vi "Durability_will_2012_07_05.vi"() -> ()   [LabVIEW 2011]
uses:
  <vilib>/DAQmx/write.llb/DAQmx Write (Counter Time 1Chan 1Samp).vi
  <vilib>/DAQmx/read.llb/DAQmx Read (Analog 1D Wfm NChan NSamp).vi
  <vilib>/measure/madcrms.llb/Basic Averaged DC-RMS for 1 Chan.vi
  <vilib>/DAQmx/miscellaneous.llb/DAQmx Fill In Error Info.vi
  <vilib>/Analysis/NI_AALBase.lvlib
  <vilib>/measure/NI_MAPro.lvlib
panel:
  out "Positive Peak":dynamicdata(graph)
  out "Negative Peak":dynamicdata(graph)
  out "Motor 1 Elapsed Time (s)":string caption="Elapsed Time Text"
  out "Motor 1 Start Time":string caption="Start Time Text"
  out "Motor 1 Down":bool
  out "Long Write":bool caption="Time has Elapsed"
  out "Short Write":bool caption="Time has Elapsed"
  out "Temps":dynamicdata(graph) caption="Signal Out"
  out "Power Graph":dynamicdata(graph) caption="Collected Signals"
  out "Errors":errorcluster
  out "RPM":dynamicdata(graph) caption="Collected Signals"
  out "Motor RPM":dbl format="%#.0f"
  out "Motor Power (watts)":dbl format="%#.4f"
  out "Power to MC1 (watts)":dbl format="%#.4f"
  out "Voltage to MC1 (volts)":dbl format="%#.4f"
  out "Current to MC1  (amps)":dbl format="%#.4f"
  in  "Manual Start":bool
  in  "Power \nSetting":i8(slide) min=0 max=100 step=10 scale=0.0..100.0
  out "Power Setting (%)":dbl format="%#.2f"
  out "Motor Temp (F)":dbl format="%.1f"
  out "Tank Temp (F)":dbl format="%.1f"
  in  "Quit 4":bool
  out "Phase to Phase Voltage":waveform(dbl)(graph)
  out "Phase Current":waveform(dbl)(graph)
  # "Temperature"
  # "MC1"
  # "Motor Power and RPM"
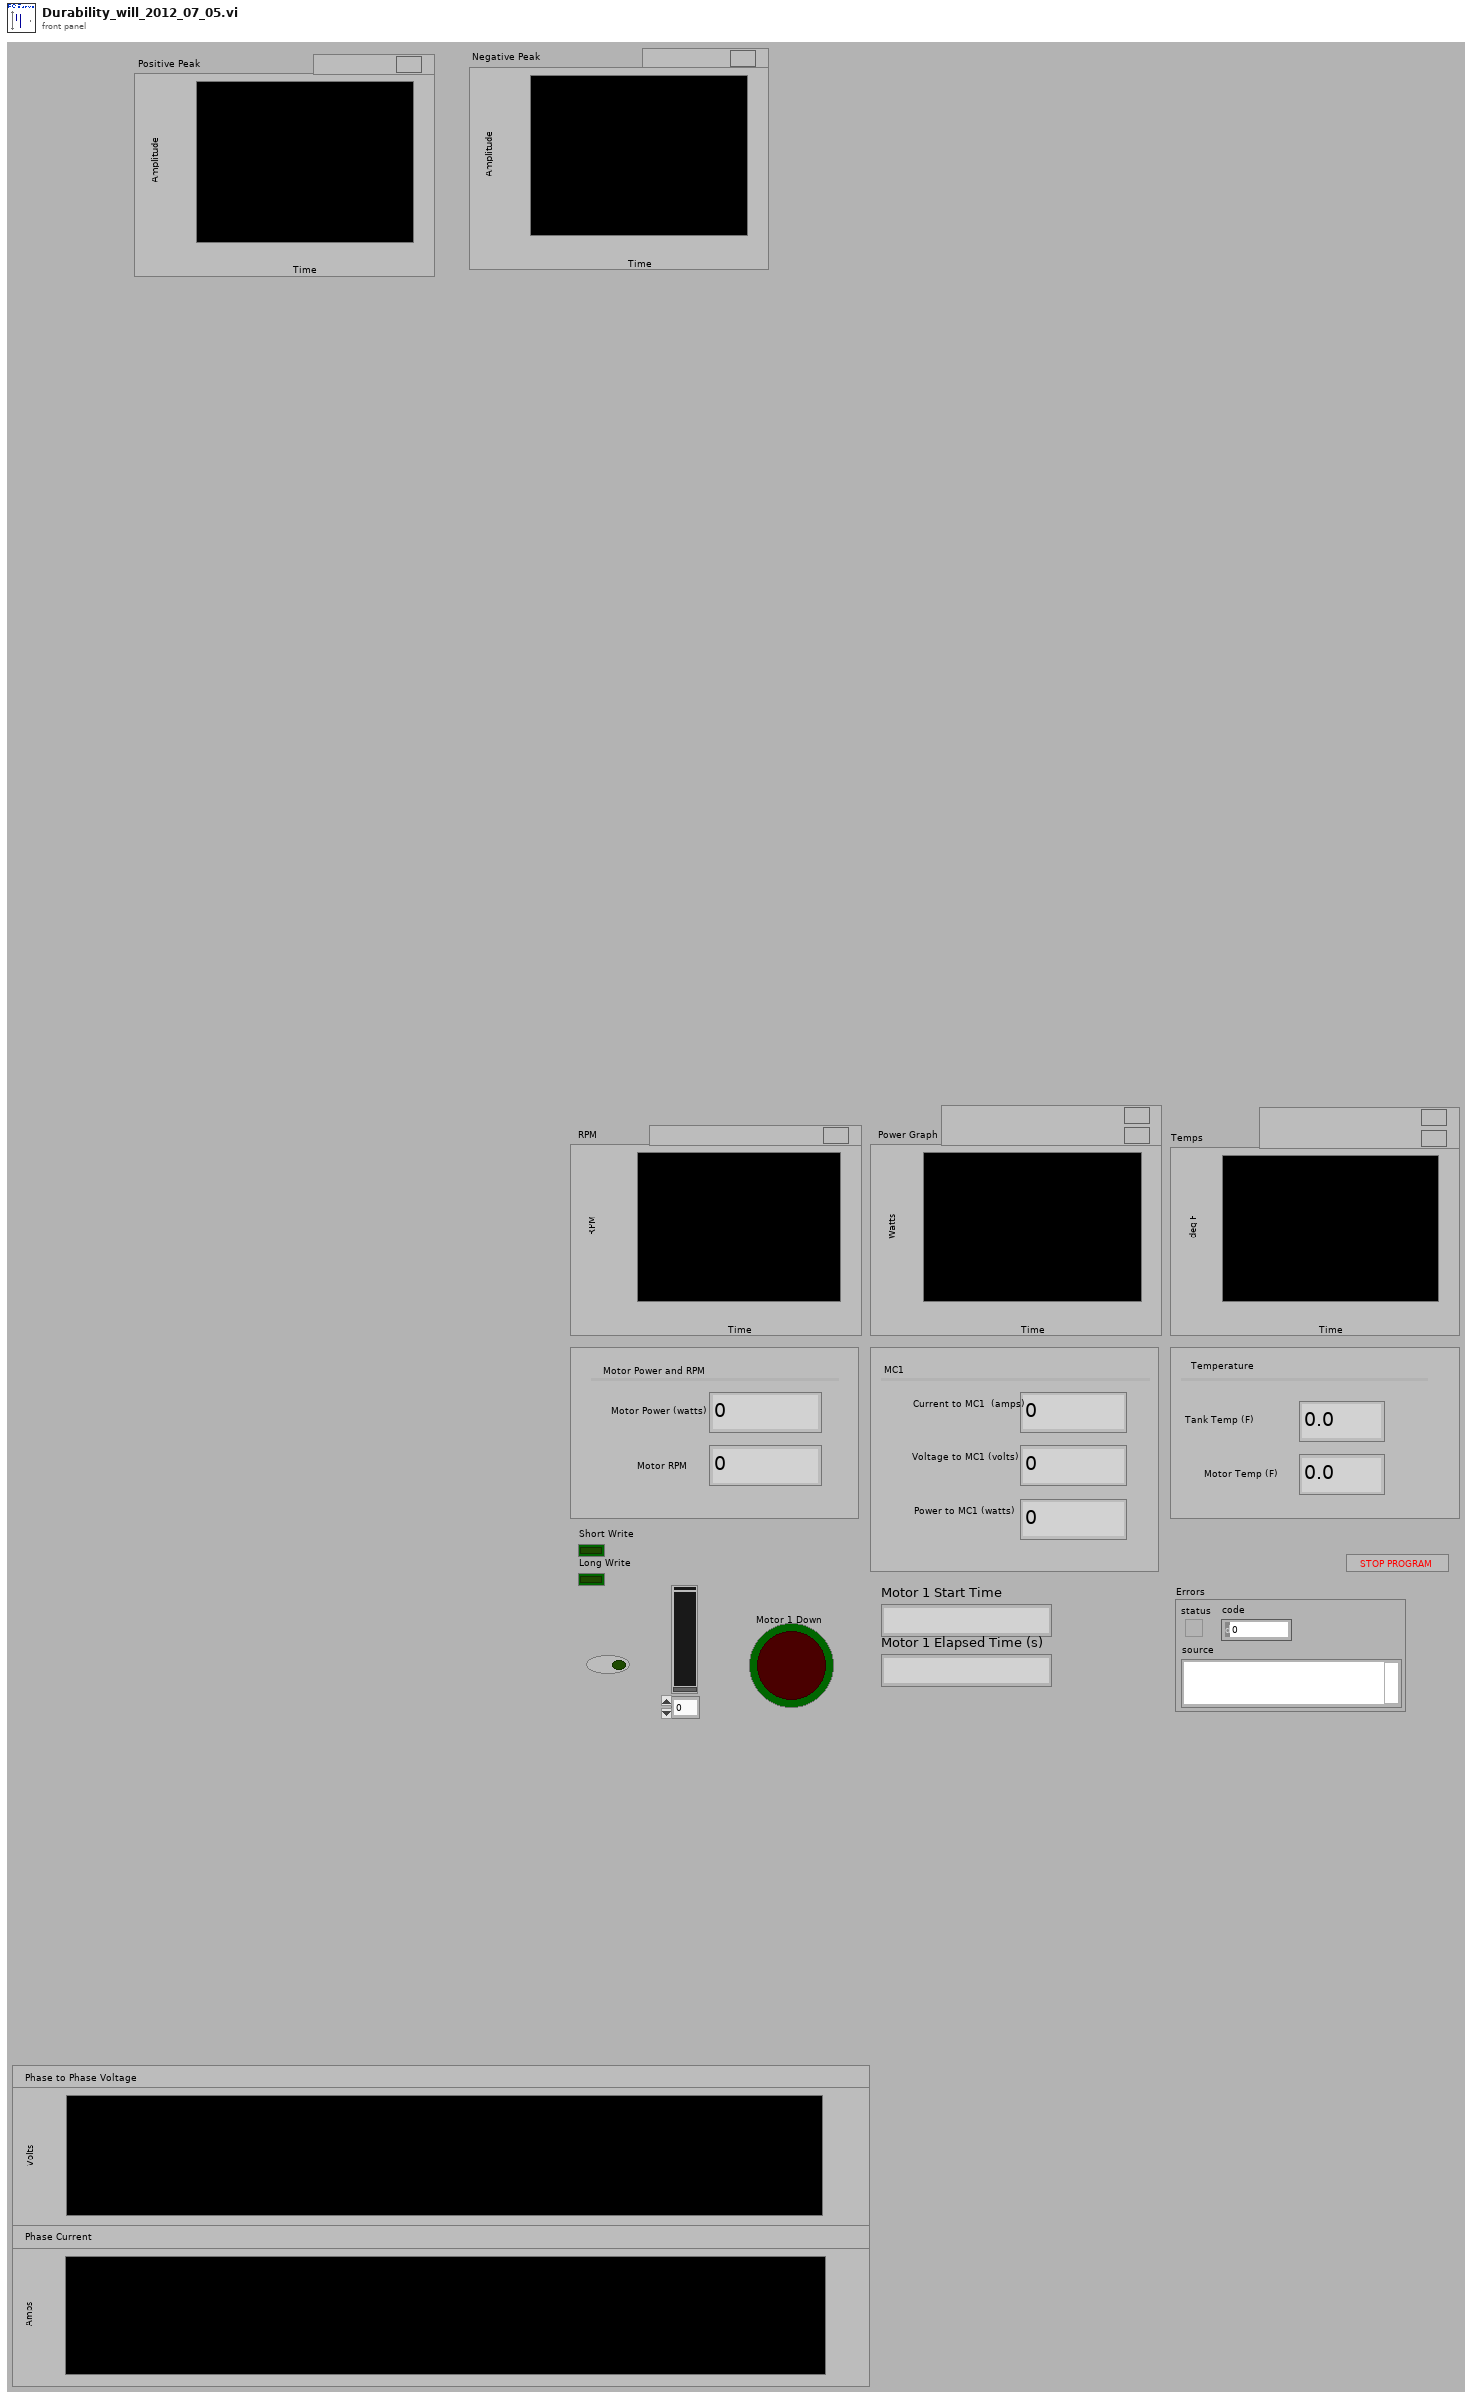
[diagram p1: front panel]
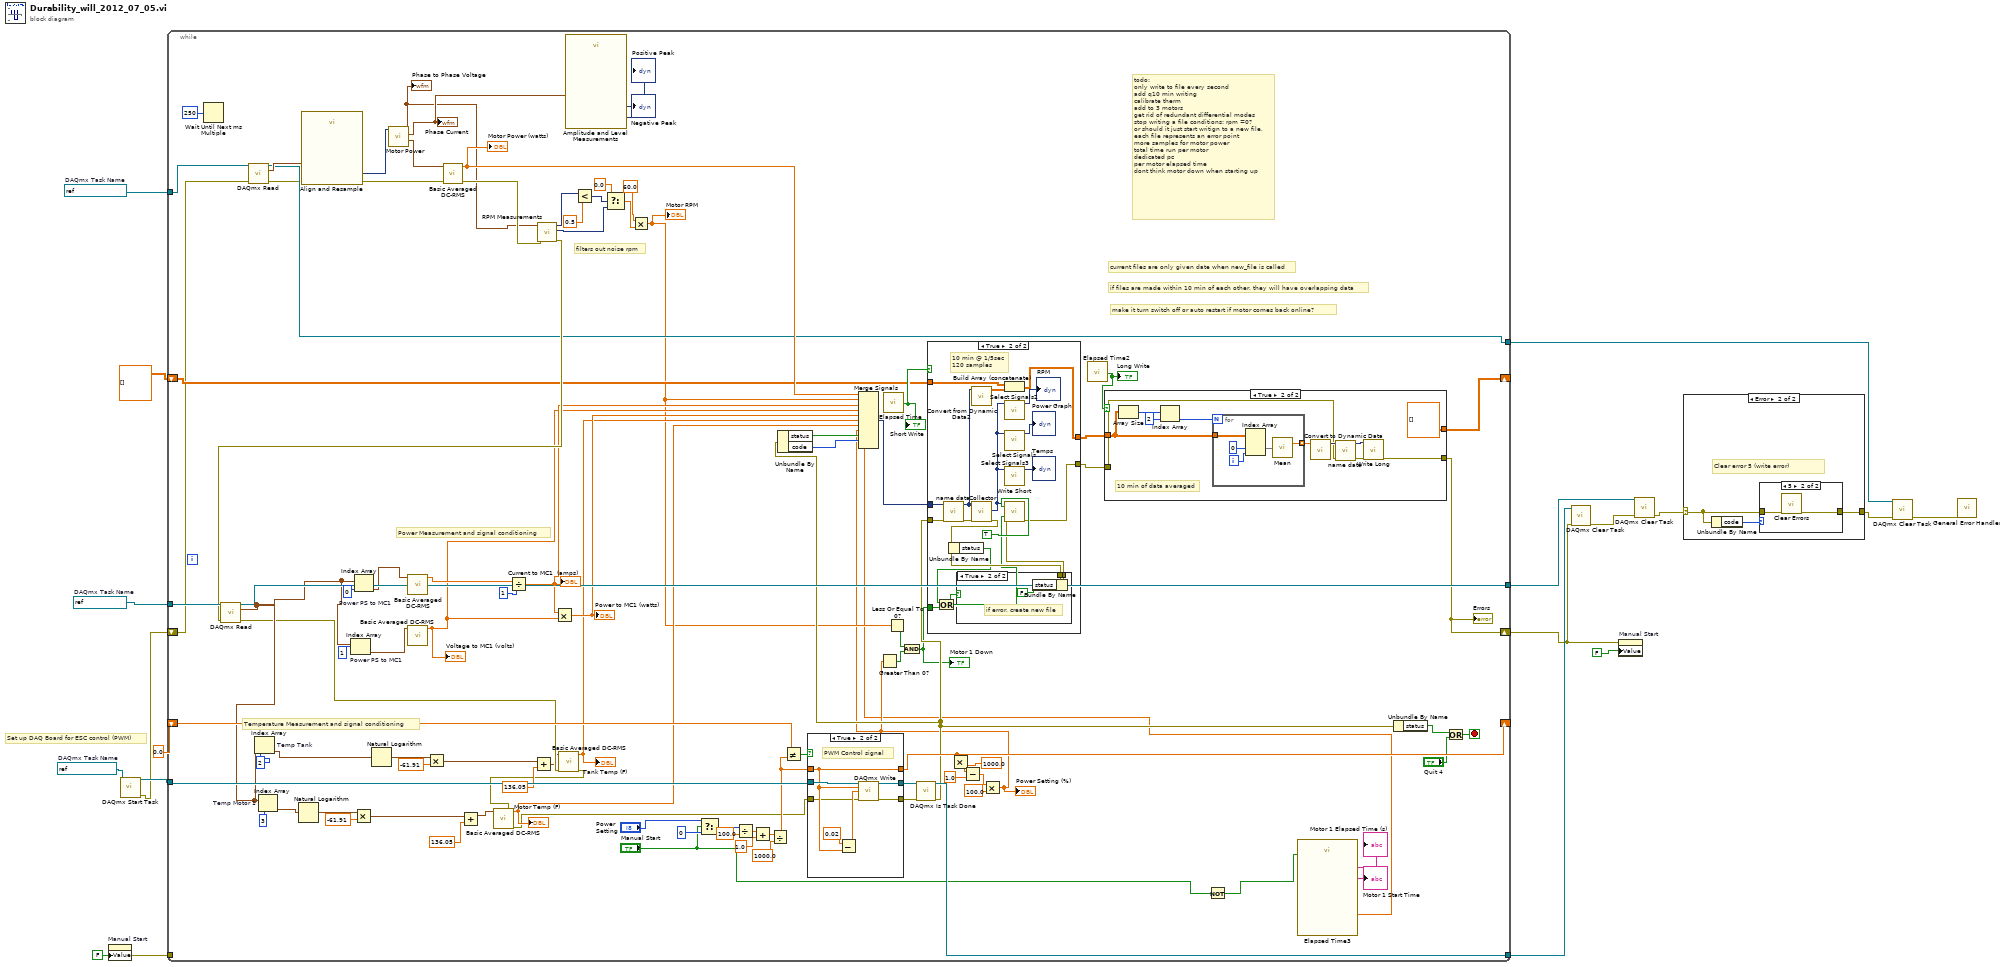
[diagram p0: block diagram]
diagram:
  w10 = refnum<k21> "PWM Signal"  # DAQmx Task Name
  w15 = refnum<k21> "MC Power"  # DAQmx Task Name
  w16 = refnum<k21> "Motor Power"  # DAQmx Task Name
  # "Set up DAQ Board for ESC control (PWM)"
  n1 = property on="Manual Start" class="Bool (strict)"("Value"=FALSE ("Run Motor")) -> (error out=w13:errorcluster)  [unwired: 2 in, 1 out]
  n2 = call <vilib>:"DAQmx Start Task.vi"("task/channels in"=w10) -> ("task out"=w9:refnum<k21>, "error out"=w1:errorcluster)  [unwired: 13 in]
  n3 = while {
    tunnel: [w115] -> w18
    tunnel: w9 -> [w113]
    shift-right: [w96] -> _
    shift-left: 0.0 -> [w104]
    tunnel: w15 -> [w91]
    tunnel: [w90] -> w17
    tunnel: [w37] -> w6
    tunnel: w16 -> [w81]
    tunnel: w13 -> [_]
    shift-right: [w40] -> _
    shift-left: dbl[][][] [] -> [w39]
    shift-right: [w36] -> w11
    shift-left: w1 -> [w33]
    stop <- w78 stop-if-true
    # "make it turn switch off or auto restart if motor comes back online?"
    # "if files are made within 10 min of each other, they will have overlapping data"
    # "current files are only given date when new_file is called"
    # "todo:\nonly write to file every second\nadd q10 min writing\ncalibrate therm\nadd to 3 motors\nget rid of redundant differential modes\nstop writing a file conditions: rpm =0?\nor should it just start writign to a new file,\neach file represents an error point\nmore samples for motor power\ntotal time run per motor\ndedicated pc\nper motor elapsed time\ndont think motor down when starting up"
    # "filters out noise rpm"
    # "Power Measurement and signal conditioning"
    # "Temperature Measurement and signal conditioning"
    n4 = Wait Until Next ms Multiple(millisecond multiple=u32 250) -> ()  [unwired: 1 out]
    n5 = call-poly <vilib>:"DAQmx Read.vi"("task/channels in"=w81, "error in"=w33) -> ("task out"=w37:refnum<k21>, "data"=w60:waveform(dbl)[], "error out"=w34:errorcluster)  [unwired: 11 in]
    n6 = call "Align and Resample"("Signals"=w60) -> ("Resampled Signals"=w61:dynamicdata)  [unwired: 8 in, 2 out]
    n7 = call "Motor Power.vi"("data"=w61) -> ("Waveform"=w55:waveform(dbl), "Phase Current"=w20:waveform(dbl), "Phase to Phase Voltage"=w19:waveform(dbl))  [unwired: 7 in, 1 out]
    "Phase Current" <- w20
    "Phase to Phase Voltage" <- w19
    n8 = call-poly <vilib>:"Basic Averaged DC-RMS.vi"("signal in"=w55) -> ("DC value"=w54:dbl)  [unwired: 7 in, 3 out]
    "Motor Power (watts)" <- w54
    n9 = call "RPM Measurements"("error in (no error)"=w34, "Signals"=w19) -> ("error out"=w77:errorcluster, "Frequency"=w85:dynamicdata, "Amplitude"=w82:dynamicdata)  [unwired: 7 in]
    n10 = call-poly <vilib>:"DAQmx Read.vi"("task/channels in"=w91, "error in"=w77) -> ("task out"=w90:refnum<k21>, "data"=w48:waveform(dbl)[], "error out"=w46:errorcluster)  [unwired: 11 in]
    n11 = Index Array "Temp Tank"(array=w48, index=2) -> (element=w49:waveform(dbl))
    n12 = Index Array "Temp Motor 1"(array=w48, index=3) -> (element=w71:waveform(dbl))
    n13 = Natural Logarithm(1:w71) -> (0:w75:waveform(dbl))
    n14 = Index Array "Power PS to MC1"(array=w48, index=1) -> (element=w51:waveform(dbl))
    n15 = Multiply(x=w75, y=-61.91) -> (x*y=w73:waveform(dbl))
    n16 = Index Array "Power PS to MC1"(array=w48, index=0) -> (element=w53:waveform(dbl))
    n17 = Natural Logarithm(1:w49) -> (0:w70:waveform(dbl))
    n18 = call-poly <vilib>:"Basic Averaged DC-RMS.vi"("signal in"=w53) -> ("DC value"=w52:dbl)  [unwired: 7 in, 3 out]
    n19 = call-poly <vilib>:"Basic Averaged DC-RMS.vi"("signal in"=w51) -> ("DC value"=w50:dbl)  [unwired: 7 in, 3 out]
    "Voltage to MC1 (volts)" <- w50
    n20 = Multiply(x=w70, y=-61.91) -> (x*y=w68:waveform(dbl))
    n21 = Add(x=w73, y=136.05) -> (x+y=w44:waveform(dbl))
    n22 = Divide(x=w52, y=1) -> (x/y=w65:dbl)
    "Current to MC1  (amps)" <- w65
    n23 = Add(x=w68, y=136.05) -> (x+y=w45:waveform(dbl))
    n24 = Multiply(x=w65, y=w50) -> (x*y=w64:dbl)
    "Power to MC1 (watts)" <- w64
    n25 = call-poly <vilib>:"Basic Averaged DC-RMS.vi"("error in (no error)"=w46, "signal in"=w45) -> ("error out"=w41:errorcluster, "DC value"=w47:dbl)  [unwired: 6 in, 2 out]
    "Tank Temp (F)" <- w47
    n26 = call-poly <vilib>:"Basic Averaged DC-RMS.vi"("error in (no error)"=w41, "signal in"=w44) -> ("error out"=w42:errorcluster, "DC value"=w43:dbl)  [unwired: 6 in, 2 out]
    "Motor Temp (F)" <- w43
    n27 = call "Amplitude and Level Measurements"("Signals"=w20) -> ("Negative Peak"=→"Negative Peak":dynamicdata, "Positive Peak"=→"Positive Peak":dynamicdata)  [unwired: 12 in, 1 out]
    n28 = Less?(x=w82, y=0.5) -> (x < y?=w84:dynamicdata)
    n29 = Select(t=0.0, s=w84, f=w85) -> (s? t:f=w87:dbl)
    n30 = Multiply(x=60.0, y=w87) -> (x*y=w32:dbl)
    "Motor RPM" <- w32
    n31 = Select(t="Power \nSetting", s="Manual Start", f=i8 0) -> (s? t:f=w102:i8)
    n32 = Divide(x=w102, y=100.0) -> (x/y=w108:dbl)
    n33 = Add(x=w108, y=1.0 ("x/y")) -> (x+y=w106:dbl)
    n34 = Divide(x=w106, y=1000.0) -> (x/y=w105:dbl)
    n35 = Not Equal?(x=w104, y=w105) -> (x != y?=w114:bool)
    n36 = case shown="True" w114 {
      tunnel: w105 -> [w159 w162]
      tunnel: w113 -> [w160 w166]
      tunnel: [w160 w164] -> w112
      tunnel: [w158 w163] -> w111
      tunnel: [w159 w162] -> w96
      tunnel: w42 -> [w158 w161]
      frame False {
      }
      frame True {
        # "PWM Control signal"
        n37 = Subtract(x=0.02, y=w162) -> (x-y=w165:dbl)
        n38 = call-poly <vilib>:"DAQmx Write.vi"("task/channels in"=w166, "high time"=w162, "low time"=w165, "error in"=w161) -> ("task out"=w164:refnum<k21>, "error out"=w163:errorcluster)  [unwired: 9 in, 1 out]
      }
    }
    n39 = call "Elapsed Time"() -> ("Time has Elapsed"=w58:bool)  [unwired: 12 in, 7 out]
    "Short Write" <- w58
    n40 = Less Or Equal To 0?(x=w32) -> (x <= 0?=w31:bool)
    n41 = call <vilib>:"DAQmx Is Task Done.vi"("task/channels in"=w112, "error in"=w111) -> ("task out"=w115:refnum<k21>, "error out"=w59:errorcluster)  [unwired: 11 in, 1 out]
    n42 = Unbundle By Name(w59) -> ("status"=w63:bool, "code"=w62:i32)
    n43 = Multiply(x=w96, y=1000.0) -> (x*y=w97:dbl)
    n44 = Subtract(x=w97, y=1.0) -> (x-y=w100:dbl)
    n45 = Multiply(x=w100, y=100.0) -> (x*y=w30:dbl)
    "Power Setting (%)" <- w30
    n46 = Greater Than 0?(x=w30) -> (x > 0?=w29:bool)
    n47 = And(x=w31, y=w29) -> (x .and. y?=w28:bool)
    "Motor 1 Down" <- w28
    n48 = call "Elapsed Time2"() -> ("Time has Elapsed"=w57:bool)  [unwired: 12 in, 7 out]
    "Long Write" <- w57
    n49 = Not(x="Manual Start") -> (.not. x?=w24:bool)
    n50 = call "Elapsed Time3"("Reset"=w24) -> ("Start Time Text"=→"Motor 1 Start Time":string, "Elapsed Time (s)"=w23:dbl, "Elapsed Time Text"=→"Motor 1 Elapsed Time (s)":string)  [unwired: 11 in, 5 out]
    n51 = Merge Signals(w54, w32, w65, w50, w64, w47, w43, w30, w63, w62, w23) -> (w56:dynamicdata)
    n52 = case shown="True" w58 {
      tunnel: w56 -> [_ w149]
      tunnel: w59 -> [w135 w146]
      tunnel: [w135 w141] -> w35
      tunnel: [w134 w153] -> w38
      tunnel: w39 -> [w134 w152]
      tunnel: w28 -> [_ w137]
      frame False {
      }
      frame True {
        # "10 min @ 1/5sec\n120 samples"
        n53 = call "name data.vi"("error in (no error)"=w146, "Dynamic Data"=w149) -> ("error out"=w147:errorcluster, "Output"=w148:dynamicdata)  [unwired: 8 in]
        n54 = call "Convert from Dynamic Data2"("Dynamic Data Type"=w148) -> ("Array"=w151:dbl[][])  [unwired: 3 in]
        n55 = call "Collector"("error in (no error)"=w147, "Signals"=w148) -> ("error out"=w139:errorcluster, "Collected Signals"=w142:dynamicdata)  [unwired: 8 in]
        n56 = Unbundle By Name(w139) -> ("status"=w138:bool)
        n57 = Or(x=w138, y=w137) -> (x .or. y?=w136:bool)
        n58 = case shown="True" w136 {
          tunnel: [w154 w157] -> w140
          tunnel: w139 -> [w154 w156]
          frame False {
          }
          frame True {
            # "if error, create new file"
            n59 = Bundle By Name(cluster=w156, "status"=FALSE) -> (w157:errorcluster)
          }
        }
        n60 = Build Array (concatenate)(w152, w151) -> (w153:dbl[][][])
        n61 = call "Select Signals2"("Signals"=w142) -> ("Signal Out"=→"RPM":dynamicdata)  [unwired: 9 in, 1 out]
        n62 = call "Select Signals"("Signals"=w142) -> ("Signal Out"=→"Power Graph":dynamicdata)  [unwired: 9 in, 1 out]
        n63 = call "Select Signals3"("Signals"=w142) -> ("Signal Out"=→"Temps":dynamicdata)  [unwired: 9 in, 1 out]
        n64 = call "Write Short"("Signals"=w142, "Reset"=TRUE, "new_file"=w136, "error in (no error)"=w140) -> ("error out"=w141:errorcluster)  [unwired: 13 in, 2 out]
      }
    }
    n65 = case shown="True" w57 {
      tunnel: w38 -> [w117 w128]
      tunnel: [w117 dbl[][][] []] -> w40
      tunnel: w35 -> [w116 w120]
      tunnel: [w116 w118] -> w36
      frame False {
      }
      frame True {
        # "10 min of data averaged"
        n66 = Array Size(array=w128) -> (size(s)=w124:i32[])
        n67 = Index Array(array=w124, index=2) -> (element=w125:i32)
        n68 = for {
          N: w125 -> [_]
          tunnel: w128 -> [w133]
          tunnel: [w129] -> w123 mode=indexing
          i -> [w132]
          n69 = Index Array(array=w133, index (dim 1)=0 ("disabled index (row)"), index (dim 2)=w132) -> (element=w131:dbl[])  [unwired: 1 in]
          n70 = call <vilib>:"Mean.vi"("X"=w131) -> ("mean"=w129:dbl)  [unwired: 1 out]
        }
        n71 = call "Convert to Dynamic Data"("Array"=w123) -> ("Dynamic Data Type"=w122:dynamicdata)  [unwired: 3 in]
        n72 = call "name data.vi"("error in (no error)"=w120, "Dynamic Data"=w122) -> ("error out"=w119:errorcluster, "Output"=w121:dynamicdata)  [unwired: 8 in]
        n73 = call "Write Long"("Signals"=w121, "error in (no error)"=w119) -> ("error out"=w118:errorcluster)  [unwired: 15 in, 2 out]
      }
    }
    "Errors" <- w36
    n74 = Unbundle By Name(w59) -> ("status"=w76:bool)
    n75 = Or(x=w76, y="Quit 4") -> (x .or. y?=w78:bool)
  }
  n76 = call <vilib>:"DAQmx Clear Task.vi"("task in"=w18, "error in"=w11) -> ("error out"=w2:errorcluster)  [unwired: 13 in]
  n77 = property on="Manual Start" class="Bool (strict)"(error in=w11, "Value"=FALSE ("Run Motor")) -> ()  [unwired: 1 in, 2 out]
  n78 = call <vilib>:"DAQmx Clear Task.vi"("task in"=w17, "error in"=w2) -> ("error out"=w4:errorcluster)  [unwired: 13 in]
  n79 = case shown="Error" w4 {
    selector: w4 -> [w168 w170]
    tunnel: [w168 w169] -> w3
    frame No Error {
    }
    frame Error {
      # "Clear error 5 (write error)"
      n80 = Unbundle By Name(w170) -> ("code"=w171:i32)
      n81 = case shown="5" w171 {
        tunnel: w170 -> [w172 w174]
        tunnel: [w172 w173] -> w169
        frame Default {
        }
        frame 5 {
          n82 = call <vilib>:"Clear Errors.vi"("error in (no error)"=w174) -> ("error out"=w173:errorcluster)  [unwired: 6 in]
        }
      }
    }
  }
  n83 = call <vilib>:"DAQmx Clear Task.vi"("task in"=w6, "error in"=w3) -> ("error out"=w5:errorcluster)  [unwired: 13 in]
  n84 = call <vilib>:"General Error Handler.vi"("error in (no error)"=w5) -> ()  [unwired: 10 in, 5 out]
